vi "GetProcessDefault.vi"(8 "error in (no error)":errorcluster) -> (0 "error out":errorcluster, 2 "found":bool, 3 "Logger in":refnum<class "Logger.lvclass">)   [LabVIEW 2026, in "Lumberjack.lvlib"]
uses:
  Lumberjack.lvlib
  Public/Logger.lvclass/Logger.lvclass
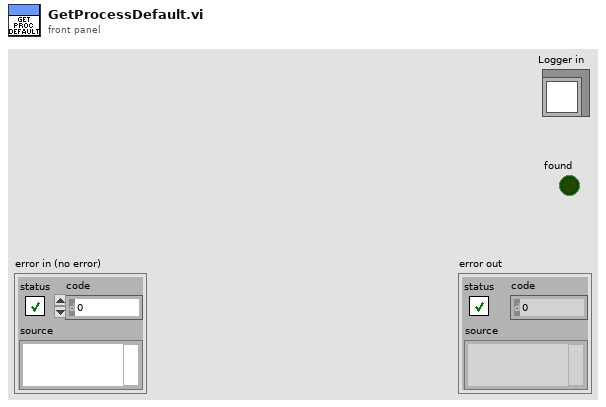
[diagram p1: front panel]
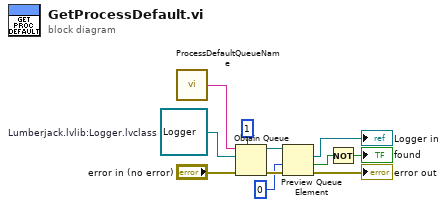
[diagram p0: block diagram]
diagram:
  w6 = refnum<class "Logger.lvclass"> refnum  # Lumberjack.lvlib:Logger.lvclass
  n1 = call "ProcessDefaultQueueName.vi"() -> ("processDefaultQueueName"=w7:string)
  n2 = Obtain Queue(max queue size (-1, unlimited)=1, name (unnamed)=w7, element data type=w6, error in (no error)="error in (no error)") -> (queue out=w8:refnum<queue>, error out=w10:errorcluster)  [unwired: 1 in, 1 out]
  n3 = Preview Queue Element(queue=w8, timeout in ms (-1)=0, error in (no error)=w10) -> (element=→"Logger in":refnum<class "Logger.lvclass">, timed out?=w3:bool, error out=→"error out":errorcluster)  [unwired: 1 out]
  n4 = Not(x=w3) -> (.not. x?=→"found":bool)
